vi "fft변환subvi.vi"(11 "배열":dbl[](array[numeric])) -> (1 "웨이브폼 그래프 4":dbl[](graph), 2 "웨이브폼 출력 2":waveform(dbl), 3 "웨이브폼 그래프 3":waveform(dbl)(graph), 4 "값 2":variant)   [LabVIEW 2015]
uses:
  <vilib>/Analysis/3filter.llb/Filter Passband Type.ctl
  <vilib>/Analysis/2dsp.llb/Real FFT.vi
  <vilib>/Analysis/3filter.llb/Butterworth Filter (DBL).vi
  <vilib>/Analysis/NI_AALPro.lvlib
  <vilib>/Analysis/NI_AALBase.lvlib
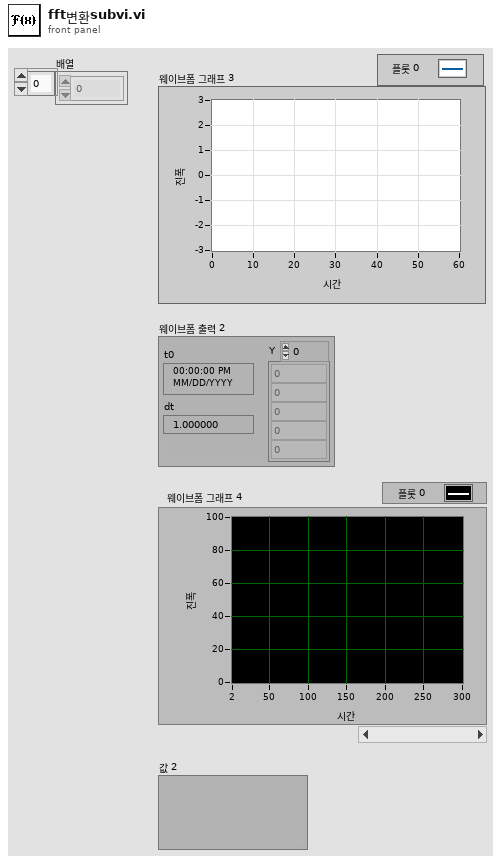
[diagram p1: front panel]
types:
  T1 = typedef "NI_AALBase.lvlib/Filter Passband Type.ctl" = enum32{"Lowpass", "Highpass", "Bandpass", "Bandstop"}
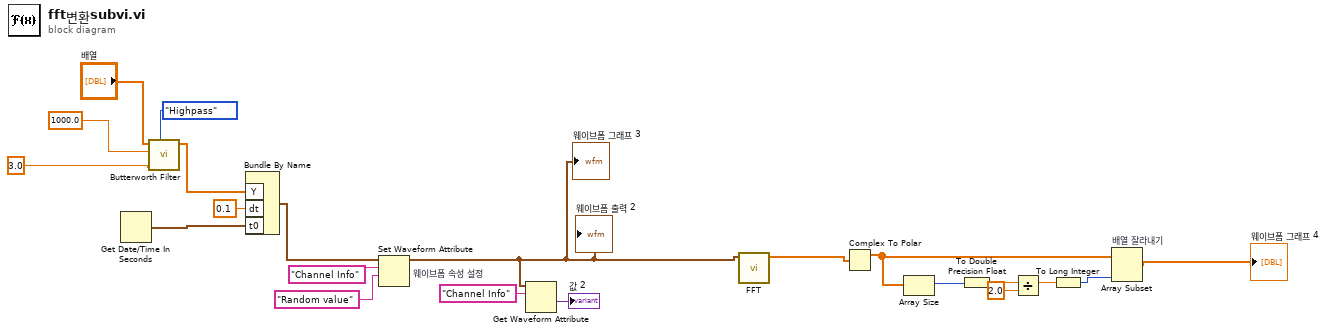
[diagram p0: block diagram]
diagram:
  n1 = Get Date/Time In Seconds() -> (seconds since 1Jan1904=w7:timestamp)
  n2 = call-poly <vilib>:"Butterworth Filter.vi"("filter type"=Filter_Passband_Type."Highpass", "low cutoff freq: fl"=3.0, "sampling freq: fs"=1000.0, "X"="배열") -> ("Filtered X"=w4:dbl[])  [unwired: 4 in, 1 out]
  n3 = Bundle By Name("Y"=w4, "dt"=0.1, "t0"=w7) -> (w8:waveform(dbl))  [unwired: 1 in]
  n4 = Set Waveform Attribute "웨이브폼 속성 설정"(5:"Random value" ("이름"), 6:"Channel Info" ("이름"), 7:w8) -> (3:w13:waveform(dbl))  [unwired: 1 in, 2 out]
  "웨이브폼 출력 2" <- w13
  "웨이브폼 그래프 3" <- w13
  n5 = Get Waveform Attribute(6:"Channel Info" ("이름"), 7:w13) -> (1:→"값 2":variant)  [unwired: 2 in, 3 out]
  n6 = call-poly <vilib>:"FFT.vi"("X"=w13) -> ("FFT {X}"=w21:cdb[])  [unwired: 9 in, 1 out]
  n7 = Complex To Polar(r * e^(i*theta)=w21) -> (r=w14:dbl[])  [unwired: 1 out]
  n8 = Array Size(array=w14) -> (size(s)=w15:i32)
  n9 = To Double Precision Float(number=w15) -> (double precision float=w16:dbl)
  n10 = Divide(x=w16, y=2.0) -> (x/y=w18:dbl)
  n11 = To Long Integer(number=w18) -> (32bit integer=w19:i32)
  n12 = Array Subset "배열 잘라내기"(array=w14, length=w19) -> (→"웨이브폼 그래프 4":dbl[])  [unwired: 1 in]
